vi "LCDL Business Logic.vi"(8 "error in":errorcluster, 11 "CaptureDetectionLoopDataIn":T1={"Captures"=path "", "Timeout"=-1, "Reset"=TRUE, "Trigger"=FALSE, "Iteration"=0, "Capture"=path ""}) -> (0 "error out":errorcluster, 2 "Latest Frame":path, 3 "CaptureDetectionLoopDataOut":T1={"Captures"=path "", "Timeout"=-1, "Reset"=TRUE, "Trigger"=FALSE, "Iteration"=0, "Capture"=path ""})   [LabVIEW 2026, in "Launcher.lvlib"]
uses:
  Launcher.lvlib
  Capture detection loop data--cluster.ctl
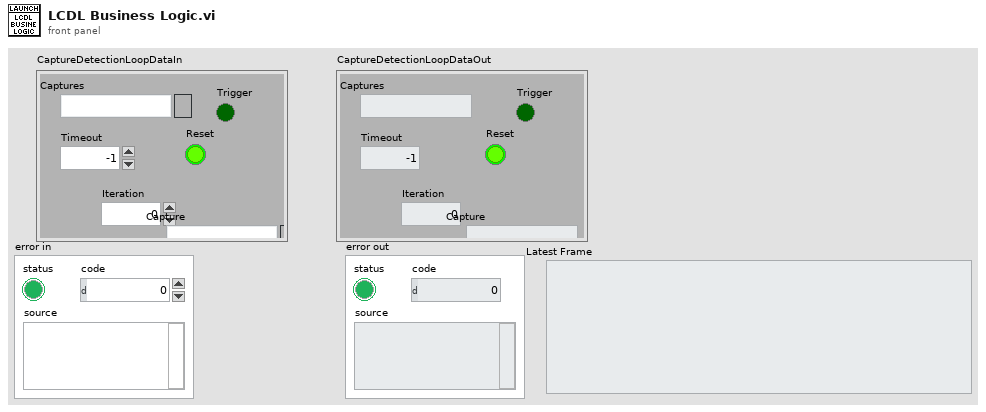
[diagram p1: front panel]
types:
  T1 = typedef "Capture detection loop data--cluster.ctl" = cluster{"Captures":path, "Timeout":i32, "Reset":bool, "Trigger":bool, "Iteration":i32, "Capture":path}
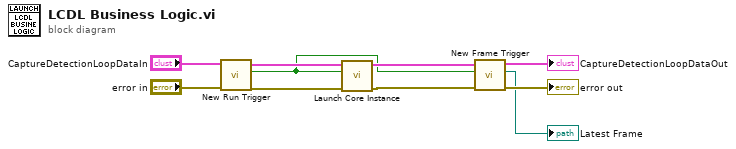
[diagram p0: block diagram]
diagram:
  n1 = call "New Run Trigger.vi"("error in"="error in", "CaptureDetectionLoopDataIn"="CaptureDetectionLoopDataIn") -> ("error out"=w5:errorcluster, "Trigger"=w1:bool, "CaptureDetectionLoopDataOut"=w4:T1)  [unwired: 7 in]
  n2 = call "Launch Core Instance.vi"("error in (no error)"=w5, "Trigger"=w1, "CaptureDetectionLoopDataIn"=w4) -> ("error out"=w2:errorcluster, "CaptureDetectionLoopDataOut"=w3:T1)  [unwired: 7 in]
  n3 = call "New Frame Trigger.vi"("error in"=w2, "Trigger"=w1, "CaptureDetectionLoopDataIn"=w3) -> ("error out"=→"error out":errorcluster, "Latest Frame"=→"Latest Frame":path, "CaptureDetectionLoopDataOut"=→"CaptureDetectionLoopDataOut":T1)  [unwired: 6 in]
